vi "SHIFTER.vi"() -> (8 "SHIFTER DATA":T1={"Exit Event"=refnum, "Terminate Error"={"status"=FALSE, "code"=0, "source"=""}, "User Parameter Controls"=[], "User Parameters"={"Name"="", "CPR Number"="", "Measuring Type "="", "Measuring Technique"="", "Measuring Limb"="", "Operator"="", "Doctor"="", "Comment"="", "AdditionalInfo"="", "RightArm"=[], "LeftArm"=[], "PalpationRight"="", "PalpationLeft"="", "Puls"=0.0, "Temp One"=0.0, "Temp Two"=0.0, "ActivityBox"=FALSE}, "System Parameters"={"Paper Running?"=FALSE, "GraphSelection"=FALSE, "Date"="", "Active Page"=""}, "Data Acquisition"={"Acquisition"=FALSE, "DAQmx Task"="", "DAQmx Error"={"status"=FALSE, "code"=0, "source"=""}, "Record number"=0.0, "RecordPath"=path "", "AcqDataRef"=refnum, "Duration"=timestamp(0 s since 1904-01-01), "Queue"=refnum, "Control?"=FALSE, "RelativeRecordPath"=path ""}, "Reference signal"={"DAQmx  Task "="", "Monitor"=FALSE, "Events"=0.0, "Time"=timestamp(0 s since 1904-01-01), "NullEvents"=0.0, "RefDataRef"=refnum, "Queue"=refnum}, "Data Process"={"SubpanelRef"=refnum, "ActiveItemTag"="", "Queue"=refnum}, "System Parameter Controls"=[], "Database"={"PatientdataRef"=refnum, "PatientdataPath"=path "", "Blue Pressure"=0.0, "Red Pressure"=0.0, "ActiveItemTag"="", "Height Adjustment"=0.0, "BluePositionArray"=[], "RedPositionArray"=[], "JournalPath"=path ""}, "MWL"={"PatientID"="", "Name"="", "DICOM Info"=path "", "DICOM Variables"=[], "Worklist"=[]}, "Control"={"Queue"=refnum, "SignalCluster"={"Pump"=TRUE, "Finger"=TRUE, "Ankle"=TRUE, "Fast Def"=TRUE, "Slow Def"=TRUE, "Init Cal"=TRUE, "Table Pres"=TRUE, "Table"=TRUE}}, "PageMenu"={"VI Reference"=refnum, "Queue"=refnum}, "Profile"={"VI Reference"=refnum, "Queue"=refnum}, "Configuration"={"VI Reference"=refnum, "Queue"=refnum}, "Acquisition"={"VI Reference"=refnum, "Queue"=refnum}, "Data"={"VI Reference"=refnum, "Queue"=refnum}, "Journal"={"VI Reference"=refnum, "Queue"=refnum}, "cRef"={"Menu"={"References"={"Stop Acq"=refnum, "MenuExit"=refnum, "MenuStartADC"=refnum, "PersonalInfoString"=refnum, "Profile"=refnum, "Configuration"=refnum, "Acquisition"=refnum, "Data"=refnum, "Journal"=refnum}}, "Profile"={"References"={"Search Patient ID"=refnum, "Name"=refnum, "CommentStr"=refnum, "Listbox Patient ID"=refnum, "ListboxDoctor"=refnum, "ListboxOperator"=refnum, "HospitalName"=refnum, "HospitalDepartment"=refnum, "HospitalAddress"=refnum, "EditHospInfo"=refnum, "Add Patient ID Btn"=refnum, "Query Worklist"=refnum}}, "Configuration"={"References"={"ListboxMeasurementArea"=refnum, "ListboxMeasurementTechnique"=refnum, "ListboxMeasurementMeth"=refnum, "ListboxRightSegmentNr"=refnum, "ListboxLeftSegmentNr"=refnum, "HeightAdjustmentInt"=refnum, "PalpationRight"=refnum, "PalpationLeft"=refnum, "ActivityBox"=refnum}, "New method"={"AddNewMeasurementBtn"=refnum, "Left Time Table"=refnum, "Right Time Table"=refnum}, "Old method"={"LeftArmPressureTable"=refnum, "RightArmPressureTable"=refnum, "SaveArmPressureBtn"=refnum, "Puls"=refnum, "TempTwo"=refnum, "TempOne"=refnum}, "Method"=""}, "Acquisition"={"References"={"SegmentAcqString"=refnum, "RingActGraph"=refnum}}, "Data"={"References"={"cmString"=refnum, "AdjustedHeight"=refnum, "Menu"=refnum, "Tangent On/Off"=refnum, "FilterControl"=refnum}}, "Journal"={"References"={"ReportSelection"=refnum, "Data"=refnum, "GenerateReport"=refnum, "Menu"=refnum, "Send To PACS"=refnum}}}, "Bluetooth"={"Queue"=refnum, "VI Reference"=refnum}})   [LabVIEW 2013, in "main.lvlib"]
uses:
  main.lvlib
  TypeDef - SHIFTER.ctl
  Dependencies.llb/Exit Event Ref.ctl
  New Design/Controls/Reference Cluster.ctl
  Dependencies.llb/TLB_Dependencies.lvlib
types:
  T1 = typedef "main.lvlib/TypeDef - SHIFTER.ctl" = cluster{"Exit Event":T2, "Terminate Error":errorcluster, "User Parameter Controls":refnum<vi>[], "User Parameters":cluster{"Name":string, "CPR Number":string, "Measuring Type ":string, "Measuring Technique":string, "Measuring Limb":string, "Operator":string, "Doctor":string, "Comment":string, "AdditionalInfo":string, "RightArm":string[][], "LeftArm":string[][], "PalpationRight":string, "PalpationLeft":string, "Puls":dbl, "Temp One":dbl, "Temp Two":dbl, "ActivityBox":bool}, "System Parameters":cluster{"Paper Running?":bool, "GraphSelection":bool, "Date":string, "Active Page":string}, "Data Acquisition":cluster{"Acquisition":bool, "DAQmx Task":refnum<k21>, "DAQmx Error":errorcluster, "Record number":dbl, "RecordPath":path, "AcqDataRef":refnum<vi>, "Duration":timestamp, "Queue":refnum<queue>, "Control?":bool, "RelativeRecordPath":path}, "Reference signal":cluster{"DAQmx  Task ":refnum<k21>, "Monitor":bool, "Events":dbl, "Time":timestamp, "NullEvents":dbl, "RefDataRef":refnum<vi>, "Queue":refnum<queue>}, "Data Process":cluster{"SubpanelRef":refnum<vi>, "ActiveItemTag":string, "Queue":refnum<queue>}, "System Parameter Controls":refnum<vi>[], "Database":cluster{"PatientdataRef":refnum<file>, "PatientdataPath":path, "Blue Pressure":dbl, "Red Pressure":dbl, "ActiveItemTag":string, "Height Adjustment":dbl, "BluePositionArray":dbl[][], "RedPositionArray":dbl[][], "JournalPath":path}, "MWL":cluster{"PatientID":string, "Name":string, "DICOM Info":path, "DICOM Variables":string[], "Worklist":string[][]}, "Control":cluster{"Queue":refnum<queue>, "SignalCluster":cluster{"Pump":bool, "Finger":bool, "Ankle":bool, "Fast Def":bool, "Slow Def":bool, "Init Cal":bool, "Table Pres":bool, "Table":bool}}, "PageMenu":cluster{"VI Reference":refnum<vi>, "Queue":refnum<queue>}, "Profile":cluster{"VI Reference":refnum<vi>, "Queue":refnum<queue>}, "Configuration":cluster{"VI Reference":refnum<vi>, "Queue":refnum<queue>}, "Acquisition":cluster{"VI Reference":refnum<vi>, "Queue":refnum<queue>}, "Data":cluster{"VI Reference":refnum<vi>, "Queue":refnum<queue>}, "Journal":cluster{"VI Reference":refnum<vi>, "Queue":refnum<queue>}, "cRef":T3, "Bluetooth":cluster{"Queue":refnum<queue>, "VI Reference":refnum<vi>}}
  T2 = typedef "main.lvlib/TLB_Dependencies.lvlib/Exit Event Ref.ctl" = refnum<user-event>
  T3 = typedef "main.lvlib/Reference Cluster.ctl" = cluster{"Menu":cluster{"References":cluster{"Stop Acq":refnum<vi>, "MenuExit":refnum<vi>, "MenuStartADC":refnum<vi>, "PersonalInfoString":refnum<vi>, "Profile":refnum<vi>, "Configuration":refnum<vi>, "Acquisition":refnum<vi>, "Data":refnum<vi>, "Journal":refnum<vi>}}, "Profile":cluster{"References":cluster{"Search Patient ID":refnum<vi>, "Name":refnum<vi>, "CommentStr":refnum<vi>, "Listbox Patient ID":refnum<vi>, "ListboxDoctor":refnum<vi>, "ListboxOperator":refnum<vi>, "HospitalName":refnum<vi>, "HospitalDepartment":refnum<vi>, "HospitalAddress":refnum<vi>, "EditHospInfo":refnum<vi>, "Add Patient ID Btn":refnum<vi>, "Query Worklist":refnum<vi>}}, "Configuration":cluster{"References":cluster{"ListboxMeasurementArea":refnum<vi>, "ListboxMeasurementTechnique":refnum<vi>, "ListboxMeasurementMeth":refnum<vi>, "ListboxRightSegmentNr":refnum<vi>, "ListboxLeftSegmentNr":refnum<vi>, "HeightAdjustmentInt":refnum<vi>, "PalpationRight":refnum<vi>, "PalpationLeft":refnum<vi>, "ActivityBox":refnum<vi>}, "New method":cluster{"AddNewMeasurementBtn":refnum<vi>, "Left Time Table":refnum<vi>, "Right Time Table":refnum<vi>}, "Old method":cluster{"LeftArmPressureTable":refnum<vi>, "RightArmPressureTable":refnum<vi>, "SaveArmPressureBtn":refnum<vi>, "Puls":refnum<vi>, "TempTwo":refnum<vi>, "TempOne":refnum<vi>}, "Method":string}, "Acquisition":cluster{"References":cluster{"SegmentAcqString":refnum<vi>, "RingActGraph":refnum<vi>}}, "Data":cluster{"References":cluster{"cmString":refnum<vi>, "AdjustedHeight":refnum<vi>, "Menu":refnum<vi>, "Tangent On/Off":refnum<vi>, "FilterControl":refnum<vi>}}, "Journal":cluster{"References":cluster{"ReportSelection":refnum<vi>, "Data":refnum<vi>, "GenerateReport":refnum<vi>, "Menu":refnum<vi>, "Send To PACS":refnum<vi>}}}
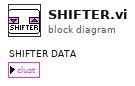
[diagram p0: block diagram]
diagram:
